vi "Load Configuration File.vi"(8 "Error In":errorcluster) -> (0 "Error Out":errorcluster, 3 "Application Configuration":T1)   [LabVIEW 2014, in "i3-docs.lvlib"]
uses:
  i3-docs.lvlib
  Controls/config.ctl
  Controls/current_config.ctl
  <vilib>/Utility/error.llb/Error Cluster From Error Code.vi
  <vilib>/Utility/config.llb/Read Key (Path).vi
  <vilib>/ErrorRing/Error Ring.xnode
  <vilib>/Utility/config.llb/NI_LVConfig.lvlib
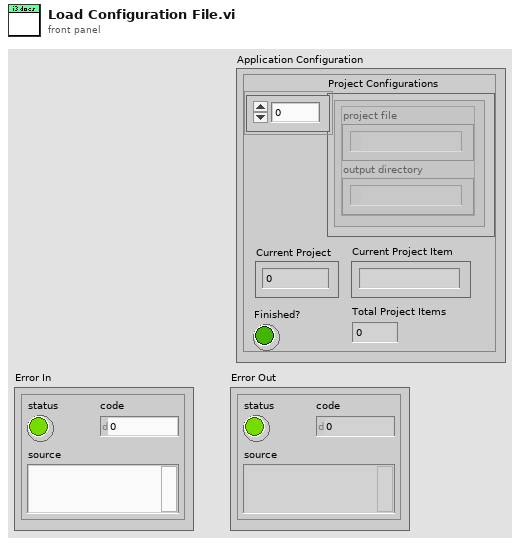
[diagram p1: front panel]
types:
  T1 = typedef "i3-docs.lvlib/config.ctl" = cluster{"Current Project":i32, "Project Configurations":T2[], "Current Project Item":string, "Finished?":bool, "Total Project Items":i32}
  T2 = typedef "i3-docs.lvlib/current_config.ctl" = cluster{"project file":path, "output directory":path}
  T3 = typedef "NI_LVConfig.lvlib/Config Data RefNum.ctl" = refnum<k1>
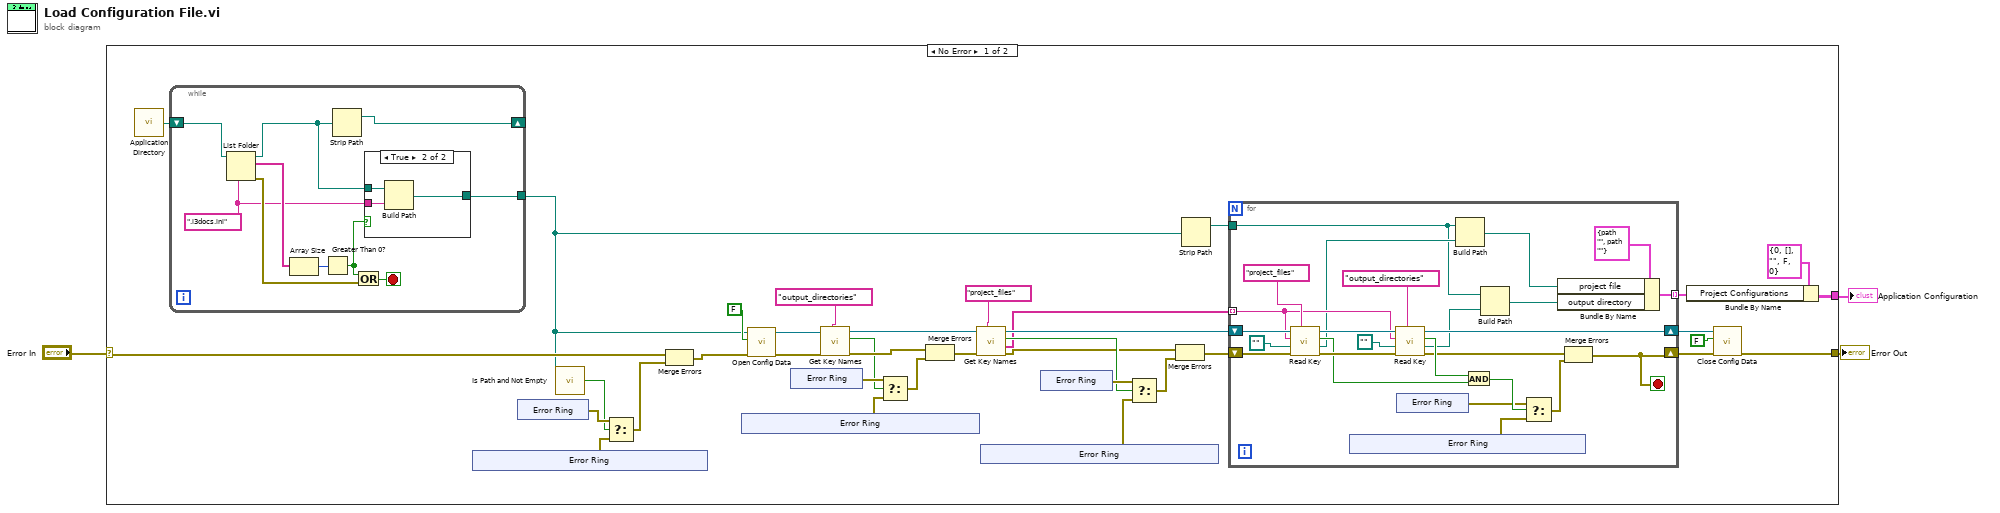
[diagram p0: block diagram]
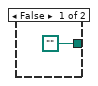
[diagram p2: hidden frame]
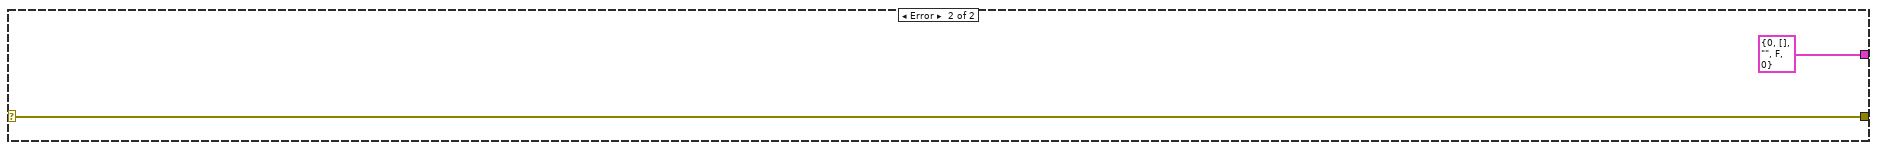
[diagram p3: hidden frame]
diagram:
  n1 = case shown="No Error" "Error In" {
    selector: "Error In" -> [w8 w104]
    tunnel: [w11 T1 {"Current Project"=0, "Project Configurations"=[], "Current Project Item"="", "Finished?"=FALSE, "Total Project Items"=0}] -> w3
    tunnel: [w7 w104] -> w1
    frame No Error {
      n2 = call <vilib>:"Application Directory.vi"() -> ("Application Directory"=w37:path)
      n3 = while {
        shift-right: [w98] -> _
        shift-left: w37 -> [w97]
        tunnel: [w89] -> w5
        stop <- w94 stop-if-true
        w91 = ".i3docs.ini" ("pattern")
        n4 = List Folder(path=w97, pattern=w91) -> (path out=w90:path, filenames=w93:string[], error out=w95:errorcluster)  [unwired: 2 in, 1 out]
        n5 = Array Size(array=w93) -> (size(s)=w96:i32)
        n6 = Greater Than 0?(x=w96) -> (x > 0?=w92:bool)
        n7 = Strip Path(path=w90) -> (stripped path=w98:path)  [unwired: 1 out]
        n8 = Or(x=w92, y=w95) -> (x .or. y?=w94:bool)
        n9 = case shown="True" w92 {
          tunnel: w91 -> [_ w101]
          tunnel: w90 -> [_ w102]
          tunnel: [path "" w100] -> w89
          frame False {
          }
          frame True {
            n10 = Build Path(base path=w102, name or relative path=w101) -> (appended path=w100:path)
          }
        }
      }
      n11 = xnode "Error Ring"() -> ("error out"=w26:errorcluster)
      n12 = xnode "Error Ring"() -> ("error out"=w25:errorcluster)
      n13 = call <vilib>:"Is Path and Not Empty.vi"("path"=w5) -> ("Is Path and Not Empty?"=w24:bool)  [unwired: 4 in]
      n14 = Select(t=w25, s=w24, f=w26) -> (s? t:f=w9:errorcluster)
      n15 = Merge Errors(w8, w9) -> (w10:errorcluster)
      n16 = xnode "Error Ring"() -> ("error out"=w31:errorcluster)
      n17 = call <vilib>:"Open Config Data.vi"("error in (no error)"=w10, "create file if necessary (T)"=FALSE, "configuration file path"=w5) -> ("error out"=w34:errorcluster, "refnum"=w36:T3)  [unwired: 6 in, 1 out]
      n18 = xnode "Error Ring"() -> ("error out"=w39:errorcluster)
      n19 = call <vilib>:"Get Key Names.vi"("section"="output_directories", "error in (no error)"=w34, "refnum"=w36) -> ("error out"=w38:errorcluster, "section exists?"=w32:bool, "refnum out"=w27:T3)  [unwired: 5 in, 1 out]
      n20 = Select(t=w39, s=w32, f=w31) -> (s? t:f=w30:errorcluster)
      n21 = Merge Errors(w38, w30) -> (w29:errorcluster)
      n22 = call <vilib>:"Get Key Names.vi"("section"="project_files", "error in (no error)"=w29, "refnum"=w27) -> ("error out"=w19:errorcluster, "key names"=w16:string[], "section exists?"=w20:bool, "refnum out"=w18:T3)  [unwired: 5 in]
      n23 = xnode "Error Ring"() -> ("error out"=w22:errorcluster)
      n24 = xnode "Error Ring"() -> ("error out"=w21:errorcluster)
      n25 = Select(t=w21, s=w20, f=w22) -> (s? t:f=w23:errorcluster)
      n26 = Merge Errors(w19, w23) -> (w17:errorcluster)
      n27 = Strip Path(path=w5) -> (stripped path=w4:path)  [unwired: 1 out]
      n28 = for {
        shift-right: [w46] -> w15
        shift-left: w17 -> [w63]
        tunnel: w16 -> [w57] mode=indexing
        shift-right: [w50] -> w14
        shift-left: w18 -> [w64]
        tunnel: [w47] -> w6 mode=indexing
        tunnel: w4 -> [w42]
        stop <- w46 stop-if-true
        n29 = call-poly <vilib>:"Read Key.vi"("section"="project_files", "error in (no error)"=w63, "default value"=path "", "key"=w57, "refnum"=w64) -> ("error out"=w59:errorcluster, "value"=w44:path, "found?"=w53:bool, "refnum out"=w60:T3)  [unwired: 3 in]
        n30 = xnode "Error Ring"() -> ("error out"=w54:errorcluster)
        n31 = call-poly <vilib>:"Read Key.vi"("section"="output_directories", "error in (no error)"=w59, "default value"=path "", "key"=w57, "refnum"=w60) -> ("error out"=w49:errorcluster, "value"=w41:path, "found?"=w52:bool, "refnum out"=w50:T3)  [unwired: 3 in]
        n32 = xnode "Error Ring"() -> ("error out"=w55:errorcluster)
        n33 = Build Path(base path=w42, name or relative path=w44) -> (appended path=w43:path)
        n34 = And(x=w52, y=w53) -> (x .and. y?=w56:bool)
        n35 = Build Path(base path=w42, name or relative path=w41) -> (appended path=w40:path)
        n36 = Select(t=w55, s=w56, f=w54) -> (s? t:f=w48:errorcluster)
        n37 = Bundle By Name(cluster=T2 {"project file"=path "", "output directory"=path ""} ("current config"), "project file"=w43, "output directory"=w40) -> (w47:T2)
        n38 = Merge Errors(w49, w48) -> (w46:errorcluster)
      }
      n39 = Bundle By Name(cluster=T1 {"Current Project"=0, "Project Configurations"=[], "Current Project Item"="", "Finished?"=FALSE, "Total Project Items"=0}, "Project Configurations"=w6) -> (w11:T1)
      n40 = call <vilib>:"Close Config Data.vi"("error in (no error)"=w15, "write file if changed (T)"=FALSE, "refnum"=w14) -> ("error out"=w7:errorcluster)  [unwired: 7 in, 1 out]
    }
    frame Error {
    }
  }
  "Error Out" <- w1
  "Application Configuration" <- w3
